vi "Init.vi"(8 "error in (no error)":errorcluster, 11 "VXMx2 in":refnum<class "VXMx2.lvclass">) -> (0 "error out":errorcluster, 3 "VXMx2 out":refnum<class "VXMx2.lvclass">)   [LabVIEW 2018, in "VXMx2.lvclass"]
uses:
  VXMx2.lvclass
  VXMx2.lvclass/VXMx2.ctl
  <instrlib>/Velmex VXM/Velmex VXM.lvlib
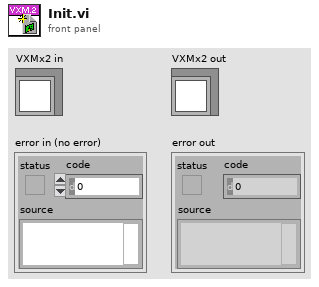
[diagram p1: front panel]
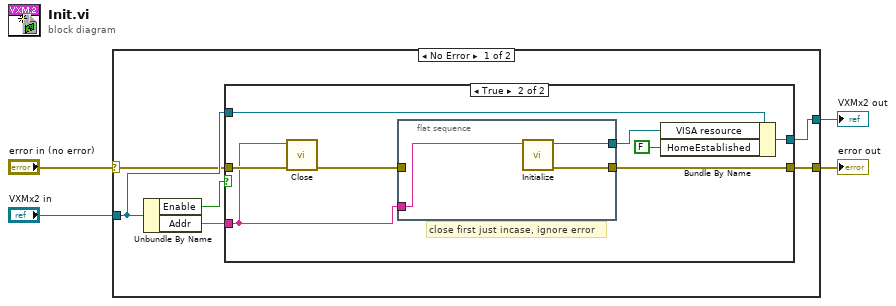
[diagram p0: block diagram]
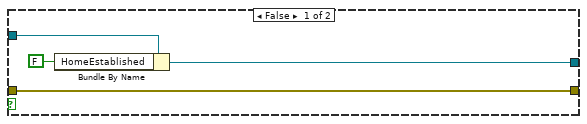
[diagram p2: hidden frame]
diagram:
  n1 = case shown="No Error" "error in (no error)" {
    selector: "error in (no error)" -> [w7 w27]
    tunnel: [w6 w27] -> w3
    tunnel: [w8 w26] -> w1
    tunnel: "VXMx2 in" -> [w10 w26]
    frame No Error {
      n2 = Unbundle By Name(w10) -> ("Enable"=w5:bool, "Addr"=w9:string)
      n3 = case shown="True" w5 {
        tunnel: w10 -> [w14 w22]
        tunnel: w9 -> [_ w16]
        tunnel: [w12 w21] -> w8
        tunnel: w7 -> [w13 w18]
        tunnel: [w13 w19] -> w6
        frame False {
          n4 = Bundle By Name(cluster=w14, "HomeEstablished"=FALSE) -> (w12:refnum<class "VXMx2.lvclass">)
        }
        frame True {
          # "close first just incase, ignore error"
          n5 = call <instrlib>:"Close.vi"("error in (no error)"=w18, "VISA resource name"=w16) -> ("error out"=w17:errorcluster)  [unwired: 9 in]
          n6 = flat-sequence {
            tunnel: w16 -> [w25]
            tunnel: [w24] -> w20
            tunnel: [w23] -> w19
            tunnel: w17 -> [_]
            frame #0 {
              n7 = call <instrlib>:"Initialize.vi"("VISA resource name"=w25) -> ("error out"=w23:errorcluster, "VISA resource out"=w24:refnum<visa-resource-name>)  [unwired: 9 in]
            }
          }
          n8 = Bundle By Name(cluster=w22, "VISA resource"=w20, "HomeEstablished"=FALSE) -> (w21:refnum<class "VXMx2.lvclass">)
        }
      }
    }
    frame Error {
    }
  }
  "error out" <- w3
  "VXMx2 out" <- w1
